vi "VI Tree - dictionary.vi"   [LabVIEW 2009]
uses:
  Dictionary Key Value Pair Cluster.ctl
panel:
  # "Dictionary VI Tree"
  # "Dictionary - VI Tree\n\nA VI that contains all of the Dictionary VIs\n\nPlease visit http://www.OpenG.org to learn about the\nOpen Source LabVIEW software movement.\n\nNOTICE -- YOU MUST LEAVE THIS NOTICE IN PLACE.  PER THE TERMS OF THE LICENSE BELOW, YOU MAY SUBLICENSE THIS SOFTWARE \nIN ANY WAY THAT DOES NOT CONFLICT WITH THIS LICENSE.\n\n### BSD License (http://www.opensource.org/licenses/bsd-license.php) Begin ###\n \nCopyright (c) 2005, Jim Kring <jim@jimkring.com>\n\nAll rights reserved.\n\nRedistribution and use in source and binary forms, with or without modification, are permitted provided that the following conditions are met:\n\n    * Redistributions of source code must retain the above copyright notice, this list of conditions and the following disclaimer.\n    * Redistributions in binary form must reproduce the above copyright notice, this list of conditions and the following disclaimer in the \n       documentation and/or other materials provided with the distribution.\n    * Neither the name of SciWare, James Kring, Inc., nor the names of its contributors may be used to endorse or promote products derived \n       from this software without specific prior written permission.\n\nTHIS SOFTWARE IS PROVIDED BY THE COPYRIGHT HOLDERS AND CONTRIBUTORS \"AS IS\" AND ANY EXPRESS OR IMPLIED WARRANTIES, \nINCLUDING, BUT NOT LIMITED TO, THE IMPLIED WARRANTIES OF MERCHANTABILITY AND FITNESS FOR A PARTICULAR PURPOSE ARE \nDISCLAIMED. IN NO EVENT SHALL THE COPYRIGHT OWNER OR CONTRIBUTORS BE LIABLE FOR ANY DIRECT, INDIRECT, INCIDENTAL,\n SPECIAL, EXEMPLARY, OR CONSEQUENTIAL DAMAGES (INCLUDING, BUT NOT LIMITED TO, PROCUREMENT OF SUBSTITUTE GOODS OR \nSERVICES; LOSS OF USE, DATA, OR PROFITS; OR BUSINESS INTERRUPTION) HOWEVER CAUSED AND ON ANY THEORY OF LIABILITY, \nWHETHER IN CONTRACT, STRICT LIABILITY, OR TORT (INCLUDING NEGLIGENCE OR OTHERWISE) ARISING IN ANY WAY OUT OF THE USE \nOF THIS SOFTWARE, EVEN IF ADVISED OF THE POSSIBILITY OF SUCH DAMAGE.\n\n### BSD License End ###"
types:
  T1 = typedef "Dictionary Key Value Pair Cluster.ctl" = cluster{"key":variant, "value":variant}
  T2 = typedef "Dictionary Object RefNum.ctl" = refnum<k1>
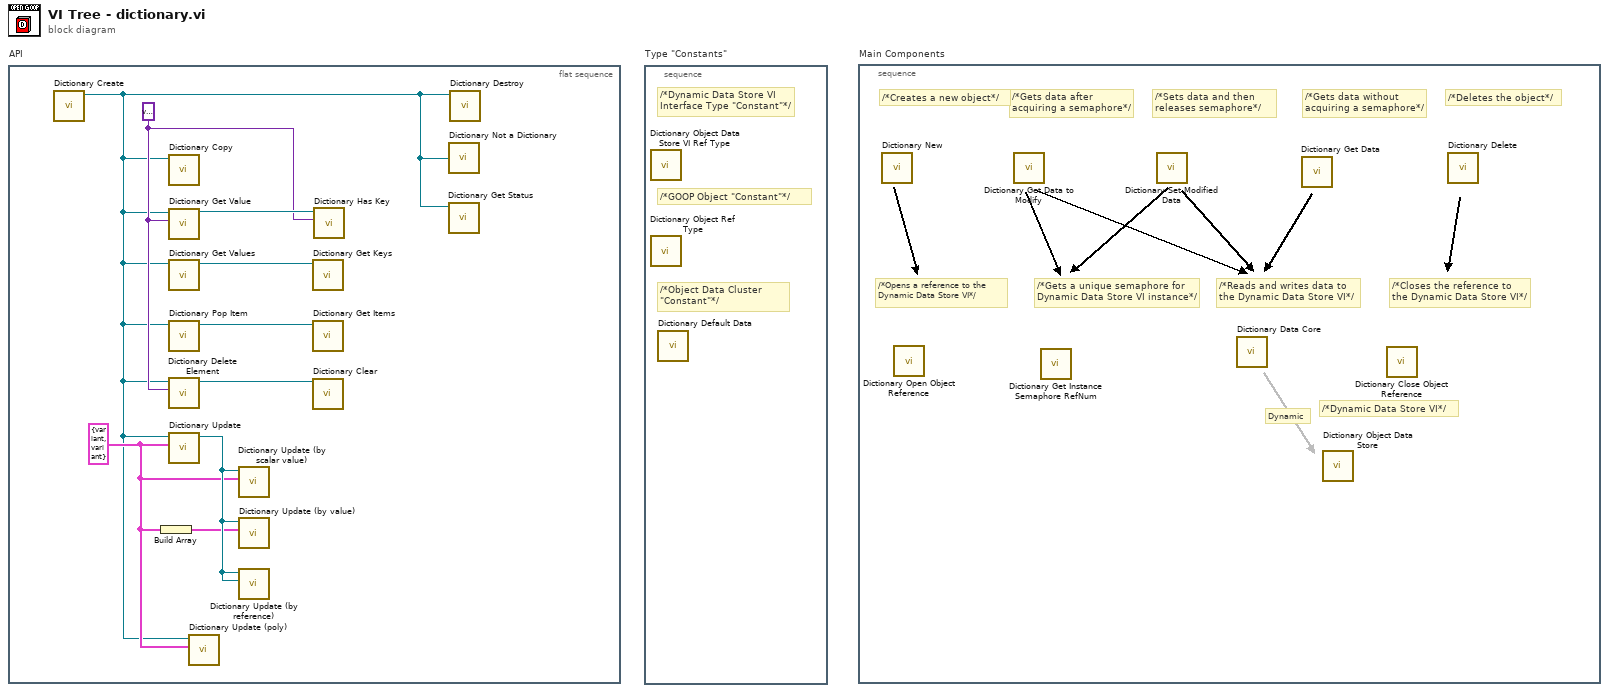
[diagram p0: block diagram]
diagram:
  n1 = flat-sequence "API" {
    frame #0 {
      w2 = T1 {"key"=variant, "value"=variant} ("key-value")
      w3 = variant ("key")
      n2 = call "Dictionary Create.vi"() -> ("dictionary out"=w1:T2)  [unwired: 10 in, 1 out]
      n3 = Build Array(w2) -> (w4:T1[])
      n4 = call "Dictionary Copy.vi"("dictionary"=w1) -> ()  [unwired: 8 in, 3 out]
      n5 = call "Dictionary Get Value.vi"("key"=w3, "dictionary"=w1) -> ("dictionary out"=w5:T2)  [unwired: 6 in, 3 out]
      n6 = call "Dictionary Get Values.vi"("dictionary"=w1) -> ("dictionary out"=w9:T2)  [unwired: 8 in, 2 out]
      n7 = call "Dictionary Pop Item.vi"("dictionary"=w1) -> ("dictionary out"=w7:T2)  [unwired: 8 in, 2 out]
      n8 = call "Dictionary Delete Element.vi"("key"=w3, "dictionary"=w1) -> ("dictionary out"=w6:T2)  [unwired: 8 in, 1 out]
      n9 = call-poly "Dictionary Update.vi"("key-value"=w2, "dictionary"=w1) -> ("dictionary out"=w8:T2)  [unwired: 7 in, 2 out]
      n10 = call-poly "Dictionary Update (poly).vi"("key-value"=w2, "dictionary"=w1) -> ()  [unwired: 7 in, 3 out]
      n11 = call "Dictionary Update (by scalar value).vi"("key-value"=w2, "dictionary"=w8) -> ()  [unwired: 7 in, 3 out]
      n12 = call "Dictionary Update (by value).vi"("dictionary with updates"=w4, "dictionary"=w8) -> ()  [unwired: 7 in, 3 out]
      n13 = call "Dictionary Update (by reference).vi"("dictionary with updates"=w8, "dictionary"=w8) -> ()  [unwired: 7 in, 3 out]
      n14 = call "Dictionary Get Keys.vi"("dictionary"=w9) -> ()  [unwired: 8 in, 3 out]
      n15 = call "Dictionary Get Items.vi"("dictionary"=w7) -> ()  [unwired: 8 in, 3 out]
      n16 = call "Dictionary Clear.vi"("dictionary"=w6) -> ()  [unwired: 9 in, 2 out]
      n17 = call "Dictionary Has Key.vi"("key"=w3, "dictionary"=w5) -> ()  [unwired: 7 in, 3 out]
      n18 = call "Dictionary Not a Dictionary.vi"("dictionary"=w1) -> ()  [unwired: 1 out]
      n19 = call "Dictionary Get Status.vi"("dictionary"=w1) -> ()  [unwired: 8 in, 3 out]
      n20 = call "Dictionary Destroy.vi"("dictionary"=w1) -> ()  [unwired: 10 in, 1 out]
    }
  }
  n21 = stacked-sequence "Type \"Constants\"" {
    frame #0 {
      # "/*Dynamic Data Store VI Interface Type \"Constant\"*/"
      # "/*GOOP Object \"Constant\"*/"
      # "/*Object Data Cluster \"Constant\"*/"
      n22 = call "Dictionary Object Data Store VI Ref Type.vi"() -> ()  [unwired: 5 in, 1 out]
      n23 = call "Dictionary Object Ref Type.vi"() -> ()  [unwired: 5 in, 1 out]
      n24 = call "Dictionary Default Data.vi"() -> ()  [unwired: 1 out]
    }
  }
  n25 = stacked-sequence "Main Components" {
    frame #0 {
      # "Dynamic"
      # "/*Opens a reference to the Dynamic Data Store VI*/"
      # "/*Reads and writes data to the Dynamic Data Store VI*/"
      # "/*Closes the reference to the Dynamic Data Store VI*/"
      # "/*Dynamic Data Store VI*/"
      # "/*Gets a unique semaphore for Dynamic Data Store VI instance*/"
      # "/*Creates a new object*/"
      # "/*Gets data after acquiring a semaphore*/"
      # "/*Sets data and then releases semaphore*/"
      # "/*Deletes the object*/"
      # "/*Gets data without acquiring a semaphore*/"
      n26 = call "Dictionary New.vi"() -> ()  [unwired: 10 in, 2 out]
      n27 = call "Dictionary Open Object Reference.vi"() -> ()  [unwired: 10 in, 2 out]
      n28 = call "Dictionary Get Data to Modify.vi"() -> ()  [unwired: 8 in, 4 out]
      n29 = call "Dictionary Get Instance Semaphore RefNum.vi"() -> ()  [unwired: 9 in, 3 out]
      n30 = call "Dictionary Set Modified Data.vi"() -> ()  [unwired: 10 in, 2 out]
      n31 = call "Dictionary Data Core.vi"() -> ()  [unwired: 9 in, 3 out]
      n32 = call "Dictionary Get Data.vi"() -> ()  [unwired: 9 in, 3 out]
      n33 = call "Dictionary Object Data Store.vi"() -> ()  [unwired: 11 in, 1 out]
      n34 = call "Dictionary Close Object Reference.vi"() -> ()  [unwired: 11 in, 1 out]
      n35 = call "Dictionary Delete.vi"() -> ()  [unwired: 11 in, 1 out]
    }
  }
